vi "Init.vi"(4 "Upload Path":path=path "", 6 "Uploads as Files?":bool=TRUE, 8 "error in (no error)":errorcluster, 9 "Stream":refnum<k5>, 11 "Request":refnum<class "Request.lvclass">) -> (0 "error out":errorcluster, 3 "Multipart Parser out":refnum<class "Multipart Parser.lvclass">)   [LabVIEW 2020, in "HTTP Utils.lvlib" / "Multipart Parser.lvclass"]
uses:
  Multipart Parser.lvclass
  Request/Request.lvclass
  Multipart Parser.lvclass/Multipart Parser.ctl
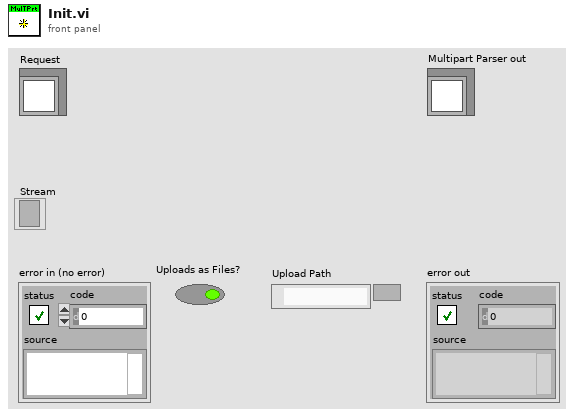
[diagram p1: front panel]
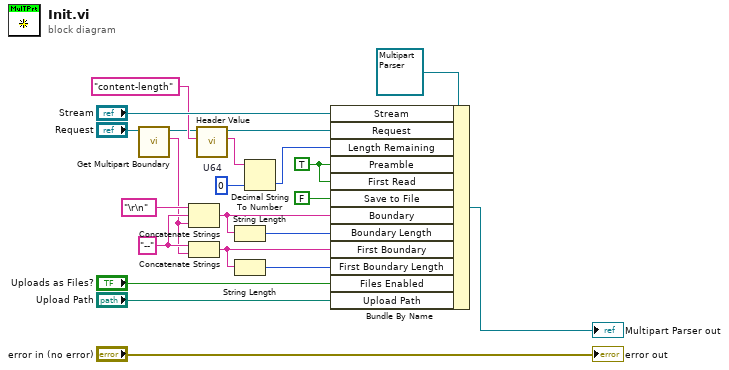
[diagram p0: block diagram]
diagram:
  w9 = "--" ("string")
  w13 = TRUE ("Preamble")
  w16 = u64 0  # U64
  n1 = call "Get Multipart Boundary.vi"("Request in"="Request") -> ("Multipart Boundary"=w6:string, "Request out"=w10:refnum<class "Request.lvclass">)  [unwired: 8 in, 1 out]
  n2 = Concatenate Strings("\r\n", w9, w6) -> (w7:string)
  n3 = Concatenate Strings(w9, w6) -> (w4:string)
  n4 = call "Header Value.vi"("Header"="content-length", "Request in"=w10) -> ("Value"=w15:string, "Request out"=w18:refnum<class "Request.lvclass">)  [unwired: 6 in, 2 out]
  n5 = String Length(string=w7) -> (length=w5:i32)
  n6 = String Length(string=w4) -> (length=w3:i32)
  n7 = Decimal String To Number(string=w15, default (0L)=w16) -> (number=w14:u64)  [unwired: 1 in, 1 out]
  n8 = Bundle By Name(cluster=refnum<class "Multipart Parser.lvclass"> refnum ("Multipart Parser in"), "Stream"="Stream", "Request"=w18, "Length Remaining"=w14, "Preamble"=w13, "First Read"=w13, "Save to File"=FALSE, "Boundary"=w7, "Boundary Length"=w5, "First Boundary"=w4, "First Boundary Length"=w3, "Files Enabled"="Uploads as Files?", "Upload Path"="Upload Path") -> (→"Multipart Parser out":refnum<class "Multipart Parser.lvclass">)
  "error out" <- "error in (no error)"
